vi "(SubVI) Delete xDNA times Force is negative.vi"(3 "xDNA":dbl[](array[numeric]), 5 "Force":dbl[](array[numeric])) -> (0 "xDNA-cut":dbl[](array[numeric]), 2 "Force-cut":dbl[](array[numeric]))   [LabVIEW 2014]
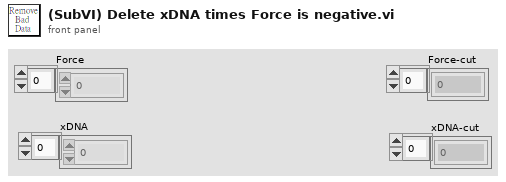
[diagram p1: front panel]
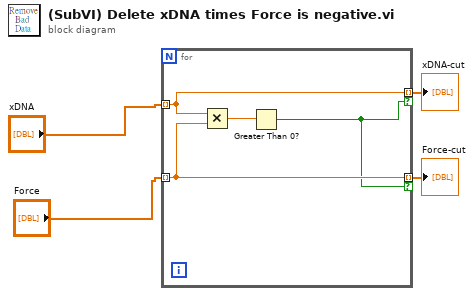
[diagram p0: block diagram]
diagram:
  n1 = for {
    tunnel: "xDNA" -> [w7] mode=indexing
    tunnel: "Force" -> [w6] mode=indexing
    tunnel: [w7] -> w2 mode=indexing if=w5
    tunnel: [w6] -> w1 mode=indexing if=w5
    n2 = Multiply(x=w7, y=w6) -> (x*y=w8:dbl)
    n3 = Greater Than 0?(x=w8) -> (x > 0?=w5:bool)
  }
  "xDNA-cut" <- w2
  "Force-cut" <- w1
